vi "pol2.vi"(9 "SerialNumber":string, 10 "position":dbl) -> (2 "GetPositionCounter":dbl)   [LabVIEW 2016]
doc: "En este subVI se controla el movimiento de la montura de rotación por medio de nodos de propiedad .NET del programa KINESIS. \n\nComo entradas tiene el número de serie del dispositivo y el ángulo al que se desea mover la montura de rotación.\nComo salidas tiene el ángulo en el que se encuentra actualmente el polarizador."
uses:
  C:/Users/Polaritones IICO/Desktop/Camara y mapeo/rot/Thorlabs.MotionControl.Controls.dll
  rot/Thorlabs.MotionControl.Controls.dll
  C:/Users/Polaritones IICO/Desktop/Camara y mapeo/rot/Thorlabs.MotionControl.IntegratedStepperMotorsCLI.dll
  rot/Thorlabs.MotionControl.IntegratedStepperMotorsCLI.dll
panel:
  in  "stop":bool
  in  "CageRotatorControl":refnum<k24>(container)
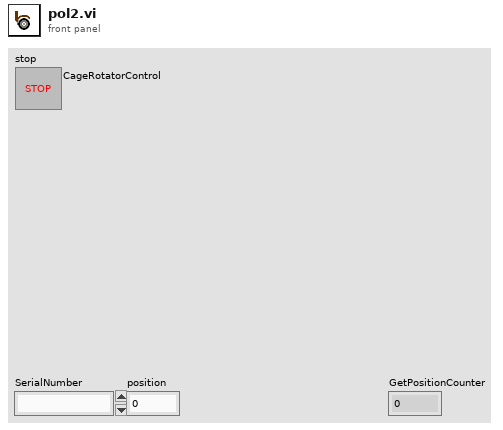
[diagram p1: front panel]
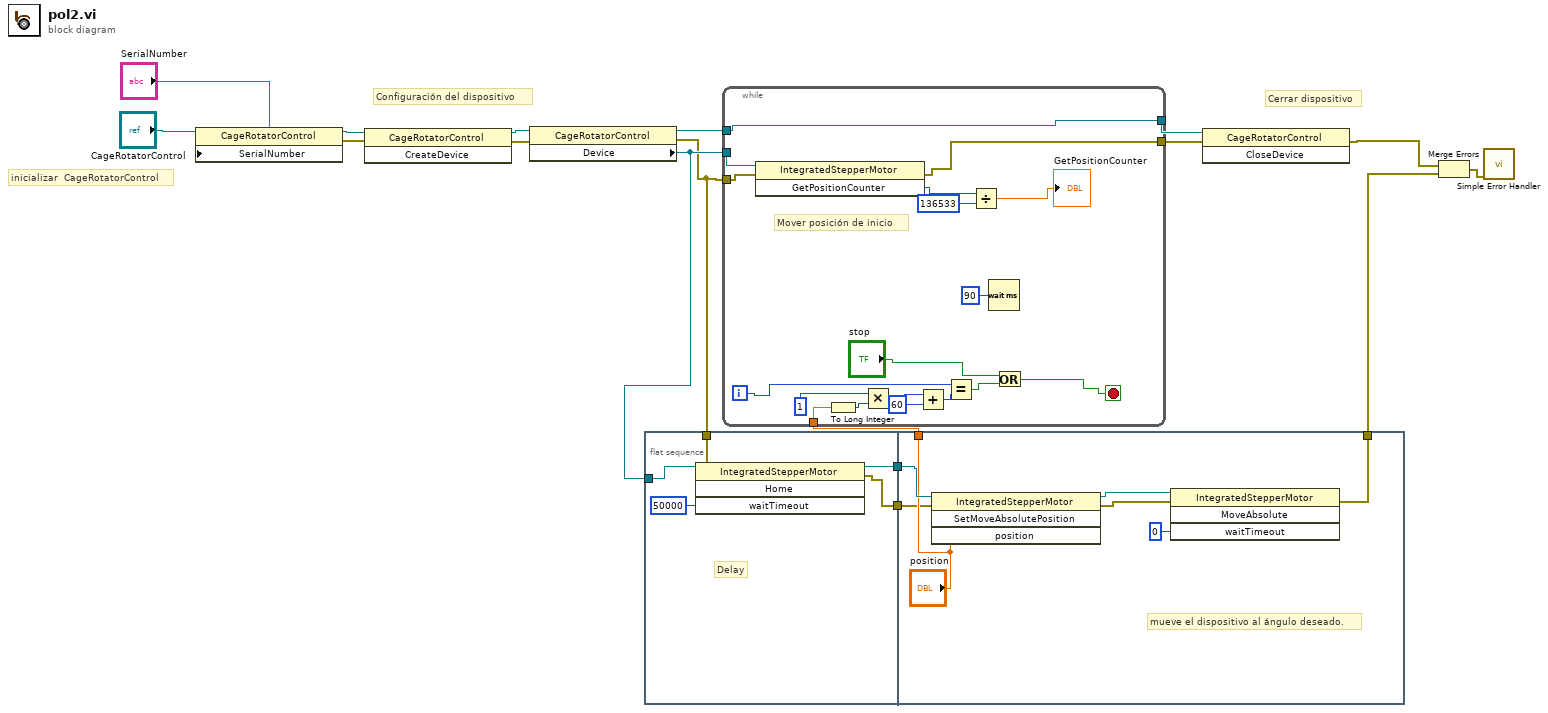
[diagram p0: block diagram]
diagram:
  # "Cerrar dispositivo"
  # "Configuración del dispositivo"
  # "inicializar  CageRotatorControl"
  n1 = property class="CageRotatorControl"(reference="CageRotatorControl", "SerialNumber"="SerialNumber") -> (reference out=w14:refnum<k24>, error out=w15:errorcluster)  [unwired: 1 in]
  n2 = invoke class="CageRotatorControl" method="CreateDevice"(reference=w14, error in=w15) -> (reference out=w12:refnum<k24>, error out=w13:errorcluster)  [unwired: 1 in, 1 out]
  n3 = property class="CageRotatorControl"(reference=w12, error in=w13) -> (reference out=w11:refnum<k24>, error out=w5:errorcluster, "Device"=w8:refnum<k24>)
  n4 = flat-sequence {
    tunnel: w8 -> [w22]
    tunnel: [w20] -> w7
    tunnel: w5 -> [w19]
    tunnel: [w18] -> w4
    tunnel: w7 -> [w29]
    tunnel: ["position"] -> w6
    tunnel: w4 -> [w25]
    tunnel: [w23] -> w2
    frame #0 {
      # "Delay"
      n5 = invoke class="IntegratedStepperMotor" method="Home"(reference=w22, error in=w19, "waitTimeout"=50000) -> (reference out=w20:refnum<k24>, error out=w18:errorcluster)  [unwired: 1 in, 2 out]
    }
    frame #1 {
      # "mueve el dispositivo al ángulo deseado."
      n6 = invoke class="IntegratedStepperMotor" method="SetMoveAbsolutePosition"(reference=w29, error in=w25, "position"="position") -> (reference out=w28:refnum<k24>, error out=w24:errorcluster)  [unwired: 1 in, 2 out]
      n7 = invoke class="IntegratedStepperMotor" method="MoveAbsolute"(reference=w28, error in=w24, "waitTimeout"=0) -> (error out=w23:errorcluster)  [unwired: 1 in, 3 out]
    }
  }
  n8 = while {
    tunnel: w8 -> [w46]
    tunnel: [w47] -> w10
    tunnel: w11 -> [w47]
    tunnel: w5 -> [w45]
    tunnel: [w44] -> w9
    tunnel: w6 -> [w31]
    i -> [w36]
    stop <- w39 stop-if-true
    # "Mover posición de inicio"
    n9 = invoke class="IntegratedStepperMotor" method="GetPositionCounter"(reference=w46, error in=w45) -> (error out=w44:errorcluster, "GetPositionCounter"=w42:i32)  [unwired: 1 in, 1 out]
    n10 = To Long Integer(number=w31) -> (32bit integer=w32:i32)
    n11 = Multiply(x=1 ("y"), y=w32) -> (x*y=w33:i32)
    n12 = Add(x=w33, y=60) -> (x+y=w34:i32)
    n13 = Equal?(x=w36, y=w34) -> (x = y?=w38:bool)
    n14 = Divide(x=w42, y=136533) -> (x/y=→"GetPositionCounter":dbl)
    n15 = Wait (ms)(milliseconds to wait=u32 90) -> ()  [unwired: 1 out]
    n16 = Or(x="stop", y=w38) -> (x .or. y?=w39:bool)
  }
  n17 = invoke class="CageRotatorControl" method="CloseDevice"(reference=w10, error in=w9) -> (error out=w3:errorcluster)  [unwired: 1 in, 2 out]
  n18 = Merge Errors(w3, w2) -> (w1:errorcluster)
  n19 = call <vilib>:"Simple Error Handler.vi"("error in (no error)"=w1) -> ()  [unwired: 4 in, 5 out]
